vi "WriteFile.vi"(8 "error in (no error)":errorcluster, 10 "data":i32[](array[numeric]), 11 "WriteOnly in":refnum<class "WriteOnly.lvclass">) -> (0 "error out":errorcluster, 3 "WriteOnly out":refnum<class "WriteOnly.lvclass">)   [LabVIEW 2021, in "WriteOnly.lvclass"]
uses:
  WriteOnly.lvclass
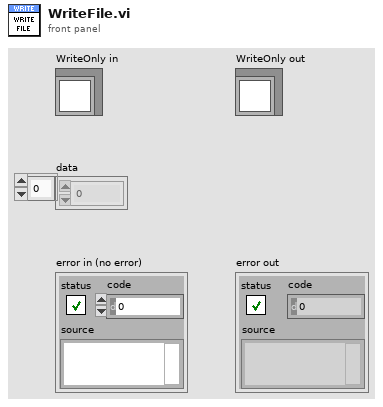
[diagram p1: front panel]
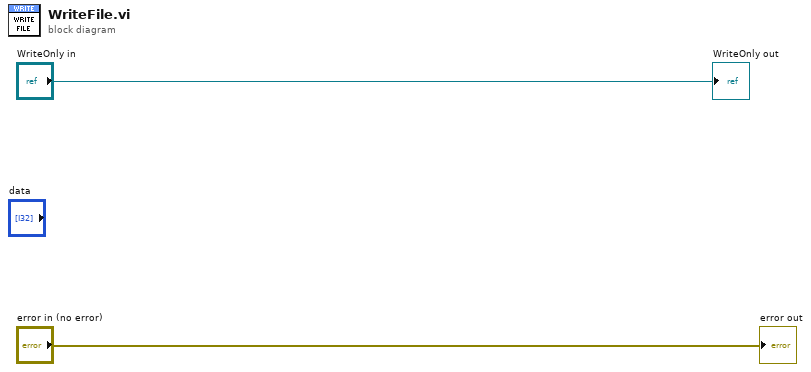
[diagram p0: block diagram]
diagram:
  "error out" <- "error in (no error)"
  "WriteOnly out" <- "WriteOnly in"
